vi "Control Motor Speed.vi"() -> ()   [LabVIEW 2016]
uses:
  <vilib>/userdefined/High Color/nirio_resource_hc.ctl
  <vilib>/FPGAPlugInAG/cRIO-9033/niLvFpga_Open_cRIO-9033.vi
  <vilib>/rvi/interface/common/dynamic/niFpgaDynamicAddResources.vi
  <vilib>/CANopenLib/CANOPEN.llb/CANopen SDO Create.vi
  Set mode of operation.vi
  Set control mode.vi
  <vilib>/rvi/interface/nirviOpenFPGA/nirviOpenFPGA.xnode
  FPGA Bitfiles/project_FPGATarget_MainFPGA_S9ZLErdeBuw.lvbitx
  FPGA/MainFPGA.vi
panel:
  in  "Motor":u8(ring) items=["Right", "Left"]
  in  "Stop":bool
  in  "Speed":i32(knob) scale=-200.0..200.0
  out "Messages sent":u16
  in  "Set":bool
  in  "error in (no error)":errorcluster
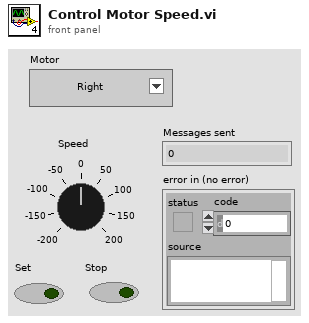
[diagram p1: front panel]
types:
  T1 = typedef "nirio_resource_hc.ctl" = tag
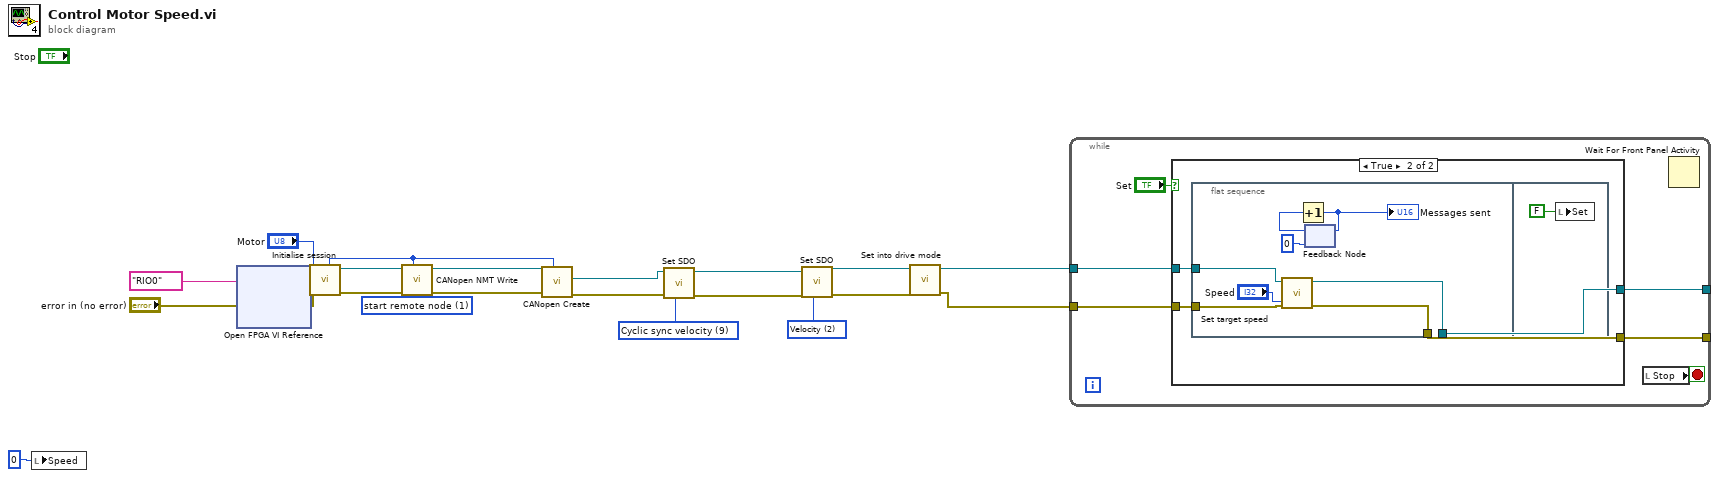
[diagram p0: block diagram]
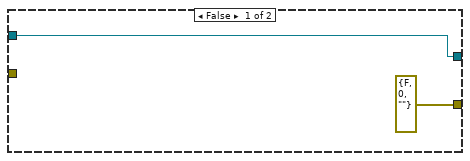
[diagram p2: hidden frame]
diagram:
  w12 = u8 2 items=["Velocity"=2, "Torque"=1] ("Control Mode")
  w13 = i8 9 items=["Induction VF – testing purposes only"=-5, "Aligning rotor position"=-4, "Current stepper – testing purposes only "=-3, "Voltage stepper – testing purposes only"=-2, "Voltage constant angle – testing purposes only"=-1, "No mode"=0, "Cyclic sync position"=8, "Cyclic sync velocity"=9, "Cyclic sync torque"=10] ("Mode of operation")
  w16 = u16 1 items=["start remote node"=1, "stop remote node"=2, "enter pre-operational"=128, "reset node"=129, "reset communication"=130] ("command")
  n1 = local write "Speed"(0 ("Speed")) -> ()
  n2 = xnode ("Open FPGA VI Reference")("error in"="error in (no error)", "resource name"=T1 "RIO0") -> ("error out"=w5:errorcluster)  [unwired: 1 out]
  n3 = call "Initialise session.vi"("error in"=w5, "Motor"="Motor") -> ("error out"=w18:errorcluster, "interface object out"=w17:refnum<k20>, "Used Node ID"=w3:u8)  [unwired: 7 in]
  n4 = call <vilib>:"CANopen NMT Write.vi"("node-ID (0)"=w3, "error in (no error)"=w18, "command"=w16, "interface object in"=w17) -> ("error out"=w15:errorcluster, "interface object out"=w14:refnum<k20>)  [unwired: 6 in]
  n5 = call-poly <vilib>:"CANopen Create.vi"("node-ID"=w3, "error in (no error)"=w15, "interface object in"=w14) -> ("error out"=w11:errorcluster, "SDO object out"=w10:refnum<k20>)  [unwired: 6 in, 1 out]
  n6 = call-poly "Set SDO.vi"("Mode of operation"=w13, "error in (no error)"=w11, "SDO object in"=w10) -> ("error out"=w8:errorcluster, "SDO object out"=w9:refnum<k20>)  [unwired: 6 in, 1 out]
  n7 = call-poly "Set SDO.vi"("Control Mode"=w12, "error in (no error)"=w8, "SDO object in"=w9) -> ("error out"=w7:errorcluster, "SDO object out"=w6:refnum<k20>)  [unwired: 6 in, 1 out]
  n8 = call "Set into drive mode.vi"("error in (no error)"=w7, "SDO object in"=w6) -> ("error out"=w2:errorcluster, "SDO object out"=w1:refnum<k20>)  [unwired: 8 in]
  n9 = while {
    tunnel: [w25] -> _
    tunnel: [w24] -> _
    tunnel: w2 -> [w23]
    tunnel: w1 -> [w22]
    stop <- w27 stop-if-true
    n10 = case shown="True" "Set" {
      tunnel: [w28 w33] -> w25
      tunnel: [errorcluster {"status"=FALSE, "code"=0, "source"=""} ("error out") w32] -> w24
      tunnel: w23 -> [_ w31]
      tunnel: w22 -> [w28 w30]
      frame False {
      }
      frame True {
        n11 = flat-sequence {
          tunnel: [w40] -> w33
          tunnel: [w39] -> w32
          tunnel: w31 -> [w35]
          tunnel: w30 -> [w34]
          frame #0 {
            n12 = call "Set target speed.vi"("Speed"="Speed", "error in (no error)"=w35, "SDO object in"=w34) -> ("error out"=w39:errorcluster, "SDO object out"=w40:refnum<k20>)  [unwired: 6 in, 1 out]
            n13 = feedback #1(u16 0) -> (w37:u16)
            n14 = Increment(x=w37) -> (x+1=w38:u16)
            "Messages sent" <- w38
            n15 = feedback-in #1(w38) -> ()
          }
          frame #1 {
            n16 = local write "Set"(FALSE ("Set")) -> ()
          }
        }
      }
    }
    n17 = local read "Stop"() -> (w27:bool)
    n18 = Wait For Front Panel Activity() -> ()  [unwired: 3 in, 1 out]
  }
